vi "ALTERA_ATP.vi"(0 "File Path Control":path=path "C:/Users/Flavio-CPGEI/Documents/ATPdata/work/Sistema_COELBA_2.atp", 5 "Condição de carga":string="0", 7 "Resistência de falta":string="0", 9 "Tipo de falta":string="0", 11 "Local de falta":string="0", 12 "Instante de falta (º)":string="0") -> (4 "path":path, 6 "Erro - chaves":bool, 8 "Erro - impedâncias":bool, 10 "Erro - string lenght":bool, 15 "error out":errorcluster)   [LabVIEW 2014]
panel:
  in  "SALVAR?":bool=TRUE
  out "substring":string
  out "index of element":i32
  out "tamanho final":i32
  out "Array inicial":i32[](array[numeric])
  out "tamanho inicial":i32
  out "Array final":i32[](array[numeric])
  out "Resistência de falta 2":string
  out "result string":string
  out "Número de cargas":i32[](array[numeric])
  in  "Resistência":string="999"
  out "IMPEDÂNCIAS":string
  in  "Ciclo em falta":string="1"
  in  "atraso":dbl=0.001431
  out "CHAVES":string
  # "Saídas"
  # "Entradas ____________________________________________________________________________"
  # "carga_redebt"
  # "carga_delta"
  # "Condições padrão ___________________________________________________________________________________________________"
  # "Instante de falta"
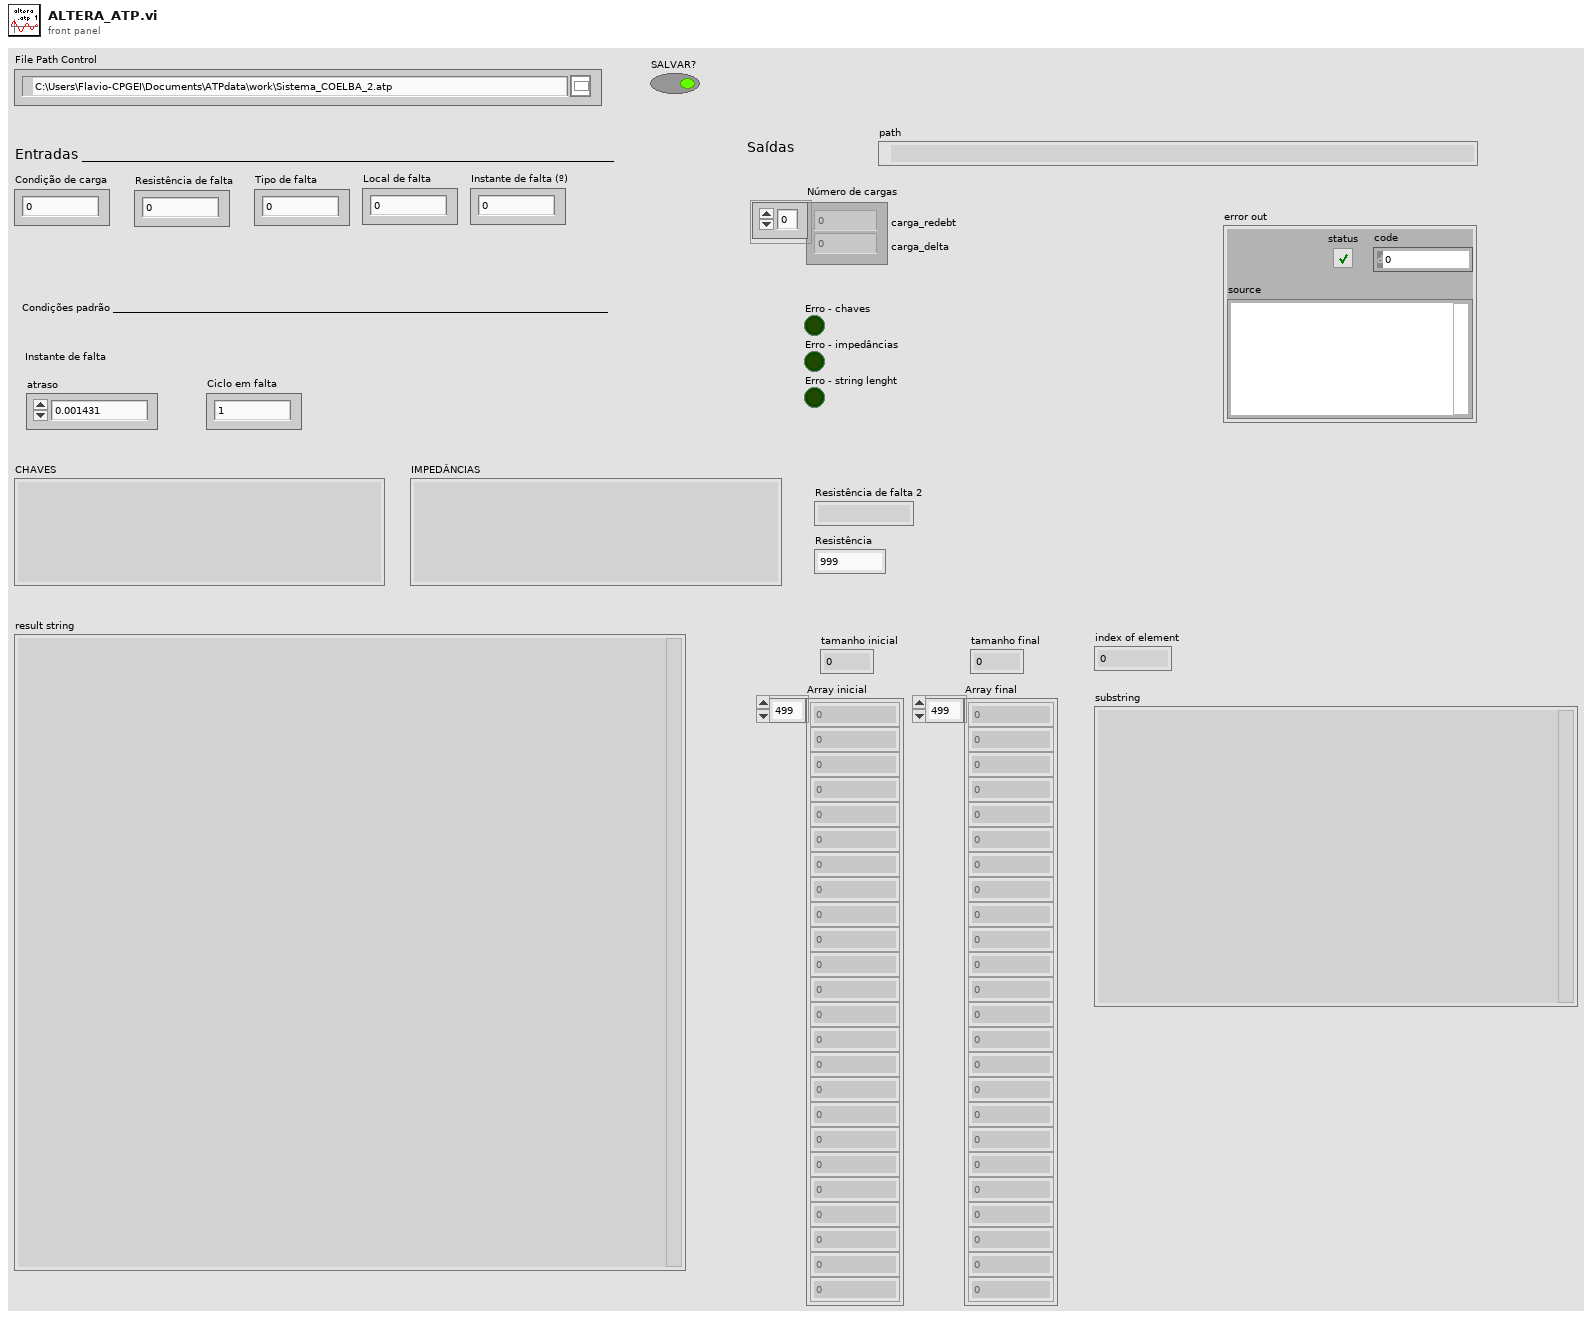
[diagram p1: front panel]
types:
  T1 = enum16{"open", "replace", "create", "open or create", "replace or create", "replace or create with confirmation"}
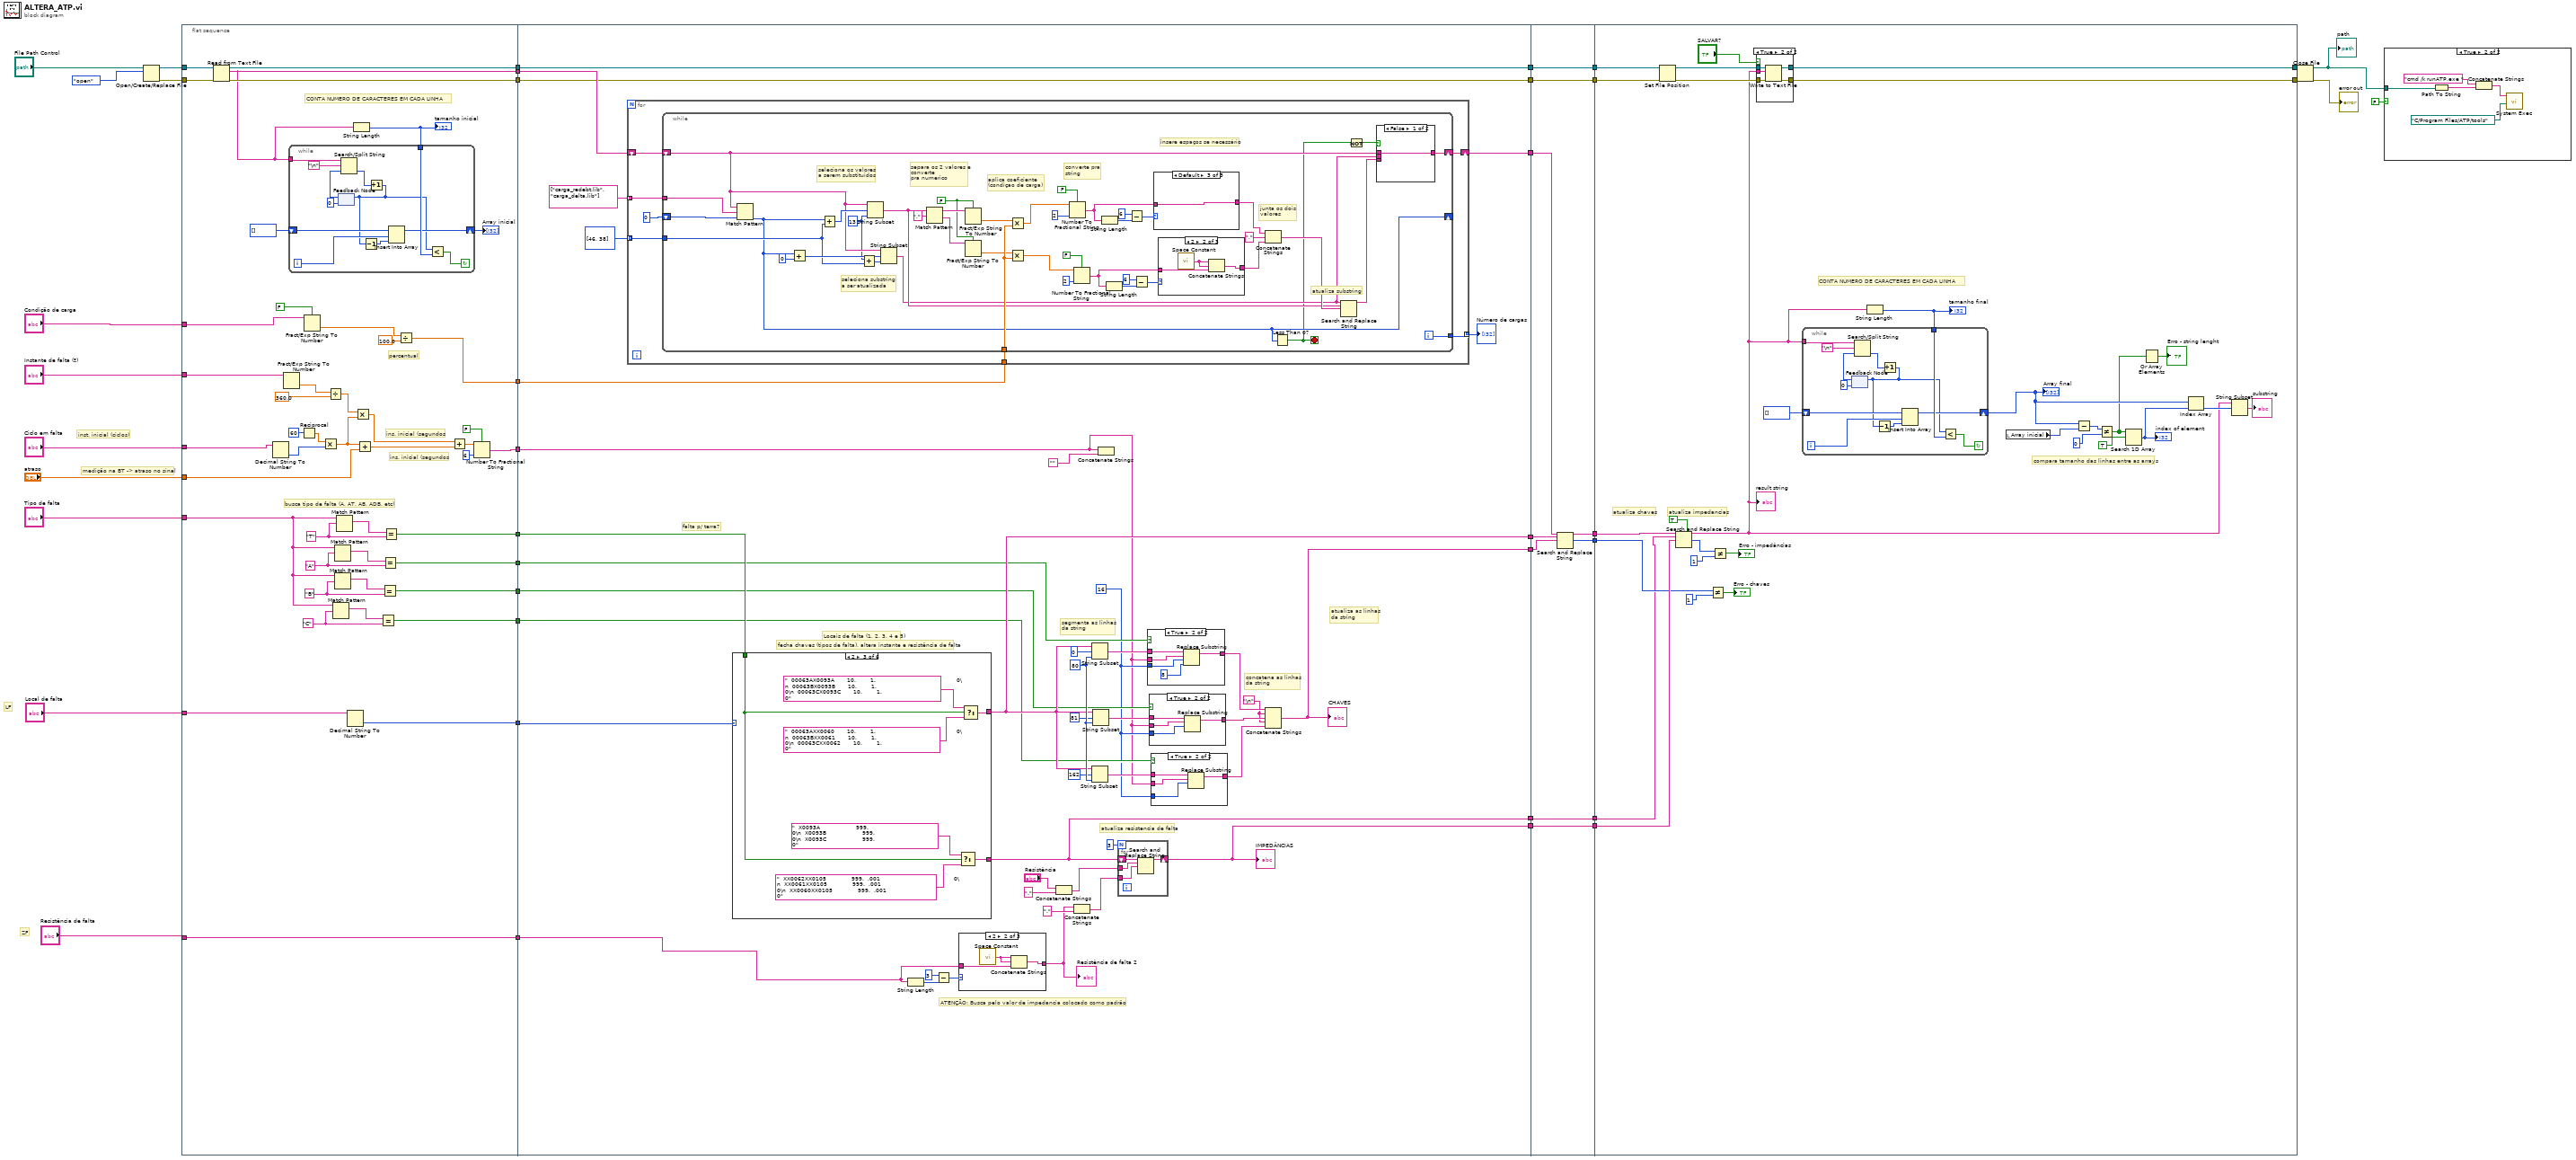
[diagram p0: block diagram]
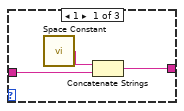
[diagram p3: hidden frame]
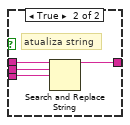
[diagram p8: hidden frame]
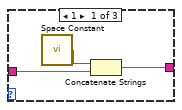
[diagram p9: hidden frame]
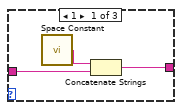
[diagram p11: hidden frame]
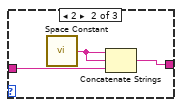
[diagram p12: hidden frame]
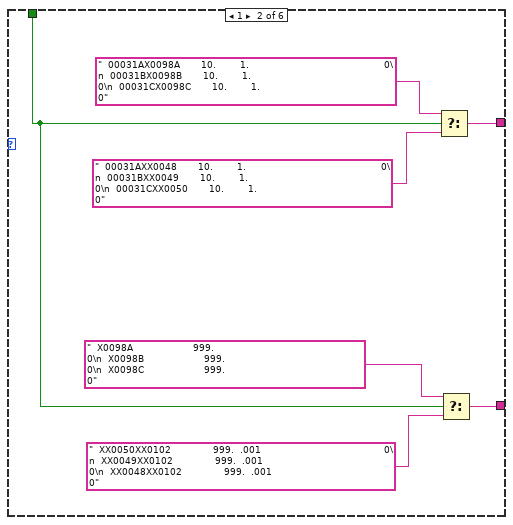
[diagram p14: hidden frame]
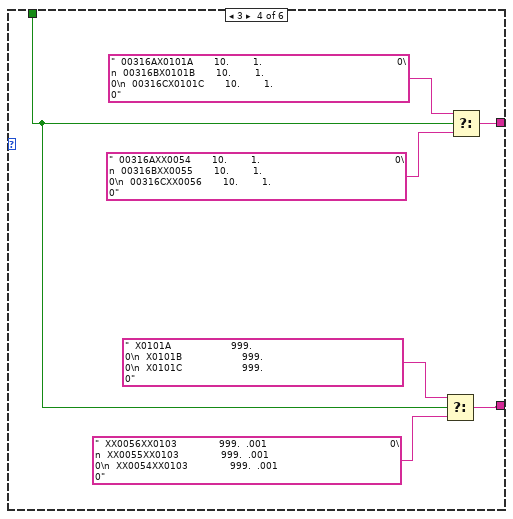
[diagram p15: hidden frame]
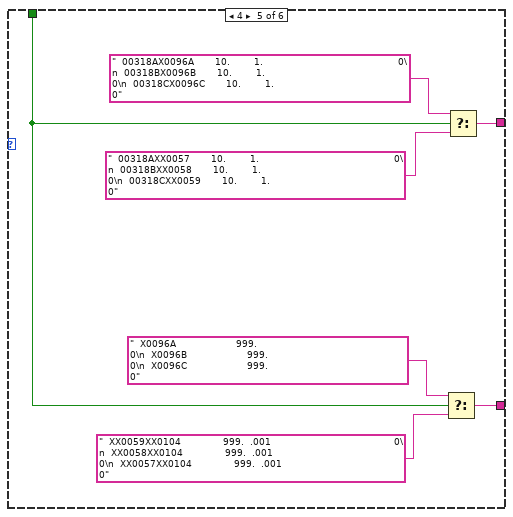
[diagram p16: hidden frame]
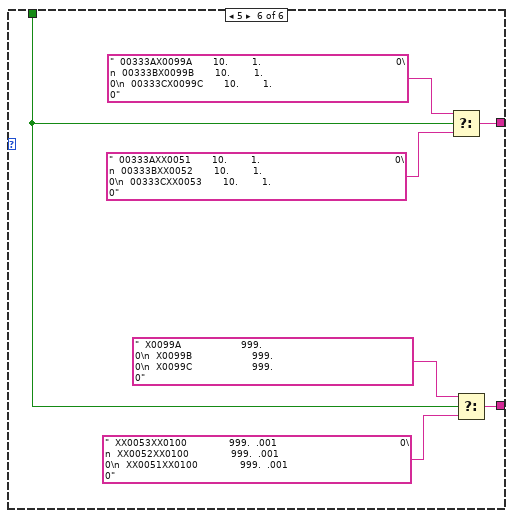
[diagram p17: hidden frame]
diagram:
  # "medição na BT -> atraso no sinal"
  # "inst. inicial (ciclos)"
  # "LF"
  # "TF"
  # "IF"
  # "ZF"
  n1 = Open/Create/Replace File(file path (use dialog)="File Path Control", operation (0:open)=T1."open") -> (refnum out=w21:refnum<file>, error out=w20:errorcluster)  [unwired: 4 in, 1 out]
  n2 = flat-sequence {
    tunnel: "Local de falta" -> [w85]
    tunnel: "Tipo de falta" -> [w71]
    tunnel: "Instante de falta (º)" -> [w67]
    tunnel: [w84] -> w40
    tunnel: [w81] -> w39
    tunnel: [w74] -> w38
    tunnel: [w73] -> w37
    tunnel: [w72] -> w36
    tunnel: [w59] -> w35
    tunnel: "Ciclo em falta" -> [w68]
    tunnel: "atraso" -> [w58]
    tunnel: [w55] -> w29
    tunnel: "Resistência de falta" -> [w55]
    tunnel: "Condição de carga" -> [w53]
    tunnel: [w46] -> w26
    tunnel: [w42] -> w25
    tunnel: [w52] -> w24
    tunnel: [w51] -> w23
    tunnel: w21 -> [w50]
    tunnel: w20 -> [w49]
    tunnel: w40 -> [w135]
    tunnel: w39 -> [w134]
    tunnel: w38 -> [w110]
    tunnel: w37 -> [w112]
    tunnel: w36 -> [w115]
    tunnel: [w116] -> w13
    tunnel: [w133] -> w12
    tunnel: w35 -> [w99]
    tunnel: w29 -> [w102]
    tunnel: w26 -> [w126]
    tunnel: [w123] -> w11
    tunnel: w25 -> [w121]
    tunnel: w24 -> [w120]
    tunnel: [w120] -> w10
    tunnel: [w119] -> w8
    tunnel: w23 -> [w119]
    tunnel: [w118] -> w6
    tunnel: [w117] -> w4
    tunnel: w13 -> [w272]
    tunnel: w12 -> [w274]
    tunnel: w11 -> [w273]
    tunnel: w10 -> [w278]
    tunnel: [w278] -> w9
    tunnel: w8 -> [w277]
    tunnel: [w277] -> w7
    tunnel: w6 -> [w276]
    tunnel: [w276] -> w5
    tunnel: w4 -> [w275]
    tunnel: [w275] -> w3
    tunnel: [w271] -> w2
    tunnel: [w270] -> w1
    tunnel: w9 -> [w303]
    tunnel: w7 -> [w305]
    tunnel: [w308] -> w19
    tunnel: [w307] -> w18
    tunnel: w5 -> [w280]
    tunnel: w3 -> [w306]
    tunnel: w2 -> [w282]
    tunnel: w1 -> [w281]
    frame #0 {
      w75 = "C" ("regular expression")
      w77 = "B" ("regular expression")
      w79 = "A" ("regular expression")
      w82 = "T" ("regular expression")
      # "percentual"
      # "CONTA NUMERO DE CARACTERES EM CADA LINHA"
      # "busca tipo de falta (A, AT, AB, ADB, etc)"
      # "ins. inicial (segundos"
      # "ins. inicial (segundos"
      n3 = Read from Text File(file (use dialog)=w50, error in=w49) -> (refnum out=w52:refnum<file>, text=w42:string, error out=w51:errorcluster)  [unwired: 2 in, 1 out]
      n4 = Decimal String To Number(string=w68) -> (number=w69:i32)  [unwired: 2 in, 1 out]
      n5 = Fract/Exp String To Number(string=w67) -> (number=w65:dbl)  [unwired: 3 in, 1 out]
      n6 = Reciprocal(x=60) -> (1/x=w70:dbl)
      n7 = Fract/Exp String To Number(use system decimal point (T)=FALSE, string=w53) -> (number=w48:dbl)  [unwired: 2 in, 1 out]
      n8 = Multiply(x=w70, y=w69) -> (x*y=w66:dbl)
      n9 = Divide(x=w65, y=360.0) -> (x/y=w63:dbl)
      n10 = Match Pattern(string=w71, regular expression=w75) -> (match substring=w76:string)  [unwired: 1 in, 3 out]
      n11 = Match Pattern(string=w71, regular expression=w77) -> (match substring=w78:string)  [unwired: 1 in, 3 out]
      n12 = Match Pattern(string=w71, regular expression=w79) -> (match substring=w80:string)  [unwired: 1 in, 3 out]
      n13 = Match Pattern(string=w71, regular expression=w82) -> (match substring=w83:string)  [unwired: 1 in, 3 out]
      n14 = Decimal String To Number(string=w85) -> (number=w84:i32)  [unwired: 2 in, 1 out]
      n15 = String Length(string=w42) -> (length=w44:i32)
      "tamanho inicial" <- w44
      n16 = while {
        tunnel: w42 -> [w96]
        shift-right: [w88] -> w43
        shift-left: i32[] [] -> [w92]
        tunnel: w44 -> [w90]
        i -> [w91]
        stop <- w89 continue-if-true
        n17 = feedback #1(0) -> (w94:i32)
        n18 = Search/Split String(string=w96, search string/char (-)="\n", offset (0)=w94) -> (offset of match=w95:i32)  [unwired: 2 out]
        n19 = Increment(x=w95) -> (x+1=w86:i32)
        n20 = feedback-in #1(w86) -> ()
        n21 = Decrement(x=w86) -> (x-1=w87:i32)
        n22 = Insert Into Array(array=w92, index=w91, new element=w87) -> (w88:i32[])
        n23 = Less?(x=w86, y=w90) -> (x < y?=w89:bool)
      }
      "Array inicial" <- w43
      n24 = Multiply(x=w63, y=w66) -> (x*y=w61:dbl)
      n25 = Add(x=w66, y=w58) -> (x+y=w62:dbl)
      n26 = Equal?(x=w76, y=w75) -> (x = y?=w72:bool)
      n27 = Equal?(x=w78, y=w77) -> (x = y?=w73:bool)
      n28 = Equal?(x=w80, y=w79) -> (x = y?=w74:bool)
      n29 = Equal?(x=w83, y=w82) -> (x = y?=w81:bool)
      n30 = Divide(x=w48, y=100.0) -> (x/y=w46:dbl)
      n31 = Add(x=w61, y=w62) -> (x+y=w60:dbl)
      n32 = Number To Fractional String(use system decimal point (T)=FALSE, number=w60, precision (6)=i16 6) -> (F-format string=w59:string)  [unwired: 1 in]
    }
    frame #1 {
      w98 = "\n"
      w108 = 16 ("offset (0)")
      w139 = 80 ("length (rest)")
      # "ATENÇÃO: Busca pelo valor de impedancia colocado como padrão"
      # "atualiza resistencia de falta"
      # "concatena as linhas\nda string"
      # "atualiza as linhas\nda string"
      # "segmenta as linhas\nda string"
      # "fecha chaves (tipos de falta), altera instante e resistência de falta"
      # "falta p/ terra?"
      # "Locais de falta (1, 2, 3, 4 e 5)"
      n33 = for {
        tunnel: w126 -> [w169]
        shift-right: [w167] -> w123
        shift-left: w121 -> [w168]
        tunnel: string[] ["carga_redebt.lib", "carga_delta.lib"] -> [w165] mode=indexing
        tunnel: i32[] [46, 38] -> [w164] mode=indexing
        tunnel: [w163] -> w122 mode=indexing
        n34 = while {
          tunnel: w169 -> [w206]
          shift-right: [w180] -> w167
          shift-left: w168 -> [w183]
          shift-right: [w172] -> _
          shift-left: 0 ("y") -> [w176]
          tunnel: w165 -> [w175]
          tunnel: w164 -> [w174]
          tunnel: [w173] -> w163
          i -> [w173]
          stop <- w170 stop-if-true
          w207 = FALSE ("use system decimal point (T)")
          w178 = 13 ("length (rest)")
          # "atualiza substring"
          # "junta os dois\nvalores"
          # "insere espaços se necessário"
          # "converte pra\nstring"
          # "aplica coeficiente\n(condiçao de carga)"
          # "separa os 2 valores e\nconverte\npra numerico"
          # "seleciona substring\na ser atualizada"
          # "seleciona os valores\na serem substituidos"
          n35 = Match Pattern(string=w183, regular expression=w175, offset (0)=w176) -> (offset past match=w172:i32)  [unwired: 3 out]
          n36 = Add(x=w172, y=0) -> (x+y=w195:i32)
          n37 = Add(x=w172, y=w174) -> (x+y=w211:i32)
          n38 = Add(x=w178, y=w174) -> (x+y=w177:i32)
          n39 = String Subset(string=w183, offset (0)=w211, length (rest)=w178) -> (substring=w182:string)
          n40 = String Subset(string=w183, offset (0)=w195, length (rest)=w177) -> (substring=w179:string)
          n41 = Match Pattern(string=w182, regular expression=",") -> (before substring=w209:string, after substring=w208:string)  [unwired: 1 in, 2 out]
          n42 = Fract/Exp String To Number(use system decimal point (T)=w207, string=w209) -> (number=w204:dbl)  [unwired: 2 in, 1 out]
          n43 = Fract/Exp String To Number(use system decimal point (T)=w207, string=w208) -> (number=w205:dbl)  [unwired: 2 in, 1 out]
          n44 = Multiply(x=w204, y=w206) -> (x*y=w203:dbl)
          n45 = Multiply(x=w205, y=w206) -> (x*y=w188:dbl)
          n46 = Number To Fractional String(use system decimal point (T)=FALSE, number=w203, precision (6)=i16 2) -> (F-format string=w197:string)  [unwired: 1 in]
          n47 = Number To Fractional String(use system decimal point (T)=FALSE, number=w188, precision (6)=i16 2) -> (F-format string=w189:string)  [unwired: 1 in]
          n48 = String Length(string=w197) -> (length=w200:i32)
          n49 = String Length(string=w189) -> (length=w192:i32)
          n50 = Subtract(x=6, y=w200) -> (x-y=w198:i32)
          n51 = Subtract(x=6, y=w192) -> (x-y=w190:i32)
          n52 = case shown="Default" w198 {
            tunnel: w197 -> [w226 w229 w230]
            tunnel: [w225 w228 w230] -> w186
            frame 1 {
              n53 = call <vilib>:"Space Constant.vi"() -> ("String"=w224:string)
              n54 = Concatenate Strings(w224, w226) -> (w225:string)
            }
            frame 2 {
              n55 = call <vilib>:"Space Constant.vi"() -> ("String"=w227:string)
              n56 = Concatenate Strings(w227, w227, w229) -> (w228:string)
            }
            frame Default {
            }
          }
          n57 = case shown="2" w190 {
            tunnel: w189 -> [w219 w222 w223]
            tunnel: [w218 w221 w223] -> w185
            frame 1 {
              n58 = call <vilib>:"Space Constant.vi"() -> ("String"=w217:string)
              n59 = Concatenate Strings(w217, w219) -> (w218:string)
            }
            frame 2 {
              n60 = call <vilib>:"Space Constant.vi"() -> ("String"=w220:string)
              n61 = Concatenate Strings(w220, w220, w222) -> (w221:string)
            }
            frame Default {
            }
          }
          n62 = Concatenate Strings(w186, "," ("regular expression"), w185) -> (w184:string)
          n63 = Less Than 0?(x=w172) -> (x < 0?=w170:bool)
          n64 = Search and Replace String(input string=w179, search string=w182, replace string=w184) -> (result string=w181:string)  [unwired: 5 in, 3 out]
          n65 = Not(x=w170) -> (.not. x?=w171:bool)
          n66 = case shown="False" w171 {
            tunnel: w183 -> [w212 w216]
            tunnel: w181 -> [_ w215]
            tunnel: [w212 w214] -> w180
            tunnel: w179 -> [_ w213]
            frame False {
            }
            frame True {
              # "atualiza string"
              n67 = Search and Replace String(input string=w216, search string=w213, replace string=w215) -> (result string=w214:string)  [unwired: 5 in, 3 out]
            }
          }
        }
      }
      "Número de cargas" <- w122
      n68 = case shown="2" w135 {
        tunnel: [_ w239 w246 w253 w260 w268] -> w116
        tunnel: w134 -> [_ w236 w242 w249 w256 w263]
        tunnel: [_ w235 w243 w250 w257 w264] -> w118
        frame Default {
        }
        frame 1 {
          n69 = Select(t="  00031AX0098A       10.        1.                                             0\n  00031BX0098B       10.        1.                                             0\n  00031CX0098C       10.        1.                                             0" ("search string"), s=w236, f="  00031AXX0048       10.        1.                                             0\n  00031BXX0049       10.        1.                                             0\n  00031CXX0050       10.        1.                                             0" ("search string")) -> (s? t:f=w239:string)
          n70 = Select(t="  X0098A                    999.                                               0\n  X0098B                    999.                                               0\n  X0098C                    999.                                               0" ("search string"), s=w236, f="  XX0050XX0102              999.  .001                                         0\n  XX0049XX0102              999.  .001                                         0\n  XX0048XX0102              999.  .001                                         0" ("search string")) -> (s? t:f=w235:string)
        }
        frame 2 {
          n71 = Select(t="  X0093A                    999.                                               0\n  X0093B                    999.                                               0\n  X0093C                    999.                                               0" ("search string"), s=w242, f="  XX0062XX0105              999.  .001                                         0\n  XX0061XX0105              999.  .001                                         0\n  XX0060XX0105              999.  .001                                         0" ("search string")) -> (s? t:f=w243:string)
          n72 = Select(t="  00063AX0093A       10.        1.                                             0\n  00063BX0093B       10.        1.                                             0\n  00063CX0093C       10.        1.                                             0" ("search string"), s=w242, f="  00063AXX0060       10.        1.                                             0\n  00063BXX0061       10.        1.                                             0\n  00063CXX0062       10.        1.                                             0" ("search string")) -> (s? t:f=w246:string)
        }
        frame 3 {
          n73 = Select(t="  X0101A                    999.                                               0\n  X0101B                    999.                                               0\n  X0101C                    999.                                               0" ("search string"), s=w249, f="  XX0056XX0103              999.  .001                                         0\n  XX0055XX0103              999.  .001                                         0\n  XX0054XX0103              999.  .001                                         0" ("search string")) -> (s? t:f=w250:string)
          n74 = Select(t="  00316AX0101A       10.        1.                                             0\n  00316BX0101B       10.        1.                                             0\n  00316CX0101C       10.        1.                                             0" ("search string"), s=w249, f="  00316AXX0054       10.        1.                                             0\n  00316BXX0055       10.        1.                                             0\n  00316CXX0056       10.        1.                                             0" ("search string")) -> (s? t:f=w253:string)
        }
        frame 4 {
          n75 = Select(t="  X0096A                    999.                                               0\n  X0096B                    999.                                               0\n  X0096C                    999.                                               0" ("search string"), s=w256, f="  XX0059XX0104              999.  .001                                         0\n  XX0058XX0104              999.  .001                                         0\n  XX0057XX0104              999.  .001                                         0" ("search string")) -> (s? t:f=w257:string)
          n76 = Select(t="  00318AX0096A       10.        1.                                             0\n  00318BX0096B       10.        1.                                             0\n  00318CX0096C       10.        1.                                             0" ("search string"), s=w256, f="  00318AXX0057       10.        1.                                             0\n  00318BXX0058       10.        1.                                             0\n  00318CXX0059       10.        1.                                             0" ("search string")) -> (s? t:f=w260:string)
        }
        frame 5 {
          n77 = Select(t="  00333AX0099A       10.        1.                                             0\n  00333BX0099B       10.        1.                                             0\n  00333CX0099C       10.        1.                                             0" ("search string"), s=w263, f="  00333AXX0051       10.        1.                                             0\n  00333BXX0052       10.        1.                                             0\n  00333CXX0053       10.        1.                                             0" ("search string")) -> (s? t:f=w268:string)
          n78 = Select(t="  X0099A                    999.                                               0\n  X0099B                    999.                                               0\n  X0099C                    999.                                               0" ("search string"), s=w263, f="  XX0053XX0100              999.  .001                                         0\n  XX0052XX0100              999.  .001                                         0\n  XX0051XX0100              999.  .001                                         0" ("search string")) -> (s? t:f=w264:string)
        }
      }
      n79 = String Length(string=w102) -> (length=w105:i32)
      n80 = Subtract(x=3, y=w105) -> (x-y=w103:i32)
      n81 = case shown="2" w103 {
        tunnel: w102 -> [w142 w145 w146]
        tunnel: [w141 w144 w146] -> w101
        frame 1 {
          n82 = call <vilib>:"Space Constant.vi"() -> ("String"=w140:string)
          n83 = Concatenate Strings(w140, w142) -> (w141:string)
        }
        frame 2 {
          n84 = call <vilib>:"Space Constant.vi"() -> ("String"=w143:string)
          n85 = Concatenate Strings(w143, w143, w145) -> (w144:string)
        }
        frame Default {
        }
      }
      "Resistência de falta 2" <- w101
      n86 = Concatenate Strings("Resistência", ".") -> (w127:string)
      n87 = Concatenate Strings(w101, ".") -> (w130:string)
      n88 = String Subset(string=w116, offset (0)=162, length (rest)=w139) -> (substring=w114:string)
      n89 = String Subset(string=w116, offset (0)=0, length (rest)=w139) -> (substring=w109:string)
      n90 = String Subset(string=w116, offset (0)=81, length (rest)=w139) -> (substring=w111:string)
      n91 = Concatenate Strings(w99, "") -> ()  [unwired: 1 out]
      n92 = for {
        N: 3 -> [_]
        tunnel: w127 -> [w233]
        shift-right: [w232] -> w117
        shift-left: w118 -> [w234]
        tunnel: w130 -> [w231]
        n93 = Search and Replace String(input string=w234, search string=w233, replace string=w231) -> (result string=w232:string)  [unwired: 5 in, 3 out]
      }
      "IMPEDÂNCIAS" <- w117
      n94 = case shown="True" w110 {
        tunnel: w109 -> [w147 w152]
        tunnel: [w147 w151] -> w107
        tunnel: w99 -> [_ w150]
        tunnel: w108 -> [_ w149]
        frame False {
        }
        frame True {
          n95 = Replace Substring(2:8 ("length (len. of substring)"), 3:w149, 4:w150, 5:w152) -> (1:w151:string)  [unwired: 1 out]
        }
      }
      n96 = case shown="True" w112 {
        tunnel: w111 -> [w153 w157]
        tunnel: [w153 w156] -> w106
        tunnel: w99 -> [_ w155]
        tunnel: w108 -> [_ w154]
        frame False {
        }
        frame True {
          n97 = Replace Substring(3:w154, 4:w155, 5:w157) -> (1:w156:string)  [unwired: 1 in, 1 out]
        }
      }
      n98 = case shown="True" w115 {
        tunnel: w114 -> [w158 w162]
        tunnel: [w158 w161] -> w113
        tunnel: w99 -> [_ w160]
        tunnel: w108 -> [_ w159]
        frame False {
        }
        frame True {
          n99 = Replace Substring(3:w159, 4:w160, 5:w162) -> (1:w161:string)  [unwired: 1 in, 1 out]
        }
      }
      n100 = Concatenate Strings(w107, w98, w106, w98, w113) -> (w133:string)
      "CHAVES" <- w133
    }
    frame #2 {
      n101 = Search and Replace String(input string=w273, search string=w272, replace string=w274) -> (result string=w271:string, number of replacements=w270:i32)  [unwired: 5 in, 2 out]
    }
    frame #3 {
      # "compara tamanho das linhas entre as arrays"
      # "CONTA NUMERO DE CARACTERES EM CADA LINHA"
      # "atualiza impedancias"
      # "atualiza chaves"
      n102 = Set File Position(refnum=w303, error in=w305) -> (refnum out=w302:refnum<file>, error out=w304:errorcluster)  [unwired: 2 in]
      n103 = Search and Replace String(multiline?=TRUE ("multiline? (F)"), input string=w282, search string=w280, replace string=w306) -> (result string=w286:string, number of replacements=w298:i32)  [unwired: 4 in, 2 out]
      "result string" <- w286
      n104 = Not Equal?(x=w281, y=1) -> (x != y?=→"Erro - chaves":bool)
      n105 = Not Equal?(x=w298, y=1) -> (x != y?=→"Erro - impedâncias":bool)
      n106 = case shown="True" "SALVAR?" {
        tunnel: [w321 w327] -> w308
        tunnel: [w322 w326] -> w307
        tunnel: w286 -> [_ w325]
        tunnel: w304 -> [w321 w324]
        tunnel: w302 -> [w322 w323]
        frame False {
        }
        frame True {
          n107 = Write to Text File(file (use dialog)=w323, text=w325, error in=w324) -> (refnum out=w326:refnum<file>, error out=w327:errorcluster)  [unwired: 1 in, 1 out]
        }
      }
      n108 = String Length(string=w286) -> (length=w299:i32)
      "tamanho final" <- w299
      n109 = while {
        tunnel: w286 -> [w319]
        shift-right: [w311] -> w288
        shift-left: i32[] [] -> [w315]
        tunnel: w299 -> [w313]
        i -> [w314]
        stop <- w312 continue-if-true
        n110 = feedback #2(0) -> (w317:i32)
        n111 = Search/Split String(string=w319, search string/char (-)="\n", offset (0)=w317) -> (offset of match=w318:i32)  [unwired: 2 out]
        n112 = Increment(x=w318) -> (x+1=w309:i32)
        n113 = feedback-in #2(w309) -> ()
        n114 = Decrement(x=w309) -> (x-1=w310:i32)
        n115 = Insert Into Array(array=w315, index=w314, new element=w310) -> (w311:i32[])
        n116 = Less?(x=w309, y=w313) -> (x < y?=w312:bool)
      }
      "Array final" <- w288
      n117 = local read "Array inicial"() -> (w293:i32[])
      n118 = Subtract(x=w288, y=w293) -> (x-y=w291:i32[])
      n119 = Not Equal?(x=w291, y=0) -> (x != y?=w284:bool[])
      n120 = Search 1D Array(1D array=w284, element=TRUE) -> (index of element=w289:i32)  [unwired: 1 in]
      "index of element" <- w289
      n121 = Or Array Elements(Boolean array=w284) -> (logical OR=→"Erro - string lenght":bool)
      n122 = Index Array(array=w288, index=w289) -> (element=w287:i32)
      n123 = String Subset(string=w286, offset (0)=w287) -> (substring=→"substring":string)  [unwired: 1 in]
    }
  }
  n124 = Close File(refnum=w18, error in=w19) -> (path=w15:path, error out=→"error out":errorcluster)
  "path" <- w15
  n125 = case shown="True" FALSE {
    tunnel: w15 -> [_ w328]
    frame False {
    }
    frame True {
      n126 = Path To String(path=w328) -> (string=w331:string)
      n127 = Concatenate Strings("cmd /k runATP.exe " ("string"), w331) -> (w329:string)
      n128 = call <vilib>:"System Exec.vi"("working directory"=path "C:/Program Files/ATP/tools", "command line"=w329) -> ()  [unwired: 6 in, 4 out]
    }
  }
